vi "ShoulderAtSetpoint.vi"(8 "SholdrSetpoints":T1=enum."ShoulderAmp") -> (0 "AtSetpoint":bool)   [LabVIEW 2023]
doc: "Makes sure the actual position of the arm is within 5 degrees of the setpoint/target"
uses:
  ShoulderGetSetpointEnum.ctl
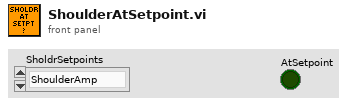
[diagram p1: front panel]
types:
  T1 = typedef "ShoulderGetSetpointEnum.ctl" = enum16{"ShoulderRest", "ShoulderShoot", "ShoulderAmp"}
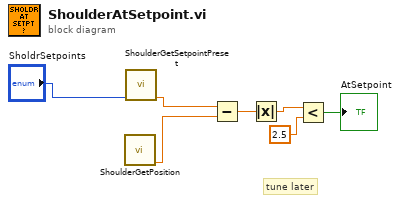
[diagram p0: block diagram]
diagram:
  # "tune later"
  n1 = call "ShoulderGetPosition.vi"() -> ("SholdrPos"=w5:dbl)  [unwired: 11 in]
  n2 = call "ShoulderGetSetpointPreset.vi"("SholdrSetpoints"="SholdrSetpoints") -> ("Setpoint"=w6:dbl)  [unwired: 10 in]
  n3 = Subtract(x=w6, y=w5) -> (x-y=w4:dbl)
  n4 = Absolute Value(x=w4) -> (abs(x)=w3:dbl)
  n5 = Less?(x=w3, y=2.5) -> (x < y?=→"AtSetpoint":bool)
